vi "S2C_FORNAX_Proc_Open.vi"(8 "Error In":errorcluster, 10 "Timeout":dbl, 11 "Data":string) -> (0 "Error Out":errorcluster, 3 "FXN_Ref":refnum<k5>)   [LabVIEW 2015]
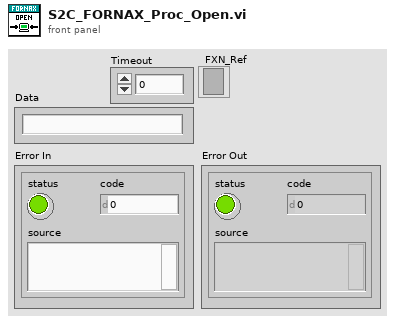
[diagram p1: front panel]
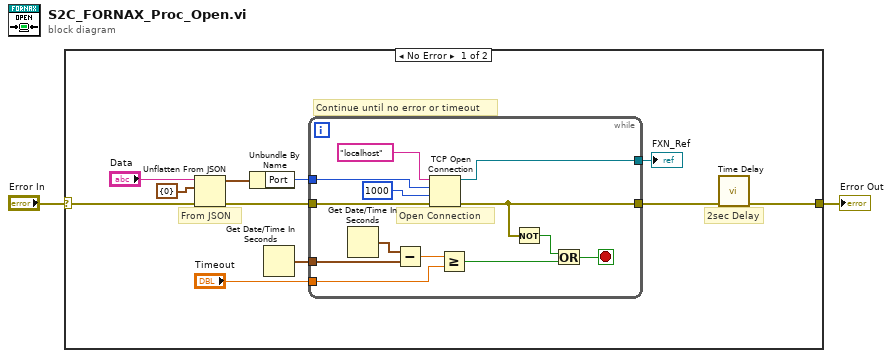
[diagram p0: block diagram]
diagram:
  n1 = case shown="No Error" "Error In" {
    selector: "Error In" -> [w6 w27]
    tunnel: [w9 w27] -> w1
    frame No Error {
      # "From JSON"
      # "2sec Delay"
      # "Continue until no error or timeout"
      n2 = Unflatten From JSON(JSON string="Data", type and defaults=cluster{"Port":u16} {"Port"=0} ("Feature Set"), error in (no error)=w6) -> (value=w7:cluster{"Port":u16}, error out=w5:errorcluster)  [unwired: 4 in]
      n3 = Unbundle By Name(w7) -> ("Port"=w4:u16)
      n4 = Get Date/Time In Seconds() -> (seconds since 1Jan1904=w13:timestamp)
      n5 = while {
        tunnel: [w24] -> w11
        tunnel: w13 -> [w20]
        tunnel: "Timeout" -> [w19]
        tunnel: w5 -> [w23]
        tunnel: [w15] -> w10
        tunnel: w4 -> [w14]
        stop <- w16 stop-if-true
        # "Open Connection"
        n6 = Get Date/Time In Seconds() -> (seconds since 1Jan1904=w21:timestamp)
        n7 = Subtract(x=w21, y=w20) -> (x-y=w22:dbl)
        n8 = TCP Open Connection(address="localhost", remote port or service name=w14, timeout ms (60000)=1000 ("timeout ms (wait forever: -1)"), error in (no error)=w23) -> (connection ID=w24:refnum<k5>, error out=w15:errorcluster)  [unwired: 1 in]
        n9 = Greater Or Equal?(x=w22, y=w19) -> (x >= y?=w17:bool)
        n10 = Not(x=w15) -> (.not. x?=w18:bool)
        n11 = Or(x=w18, y=w17) -> (x .or. y?=w16:bool)
      }
      "FXN_Ref" <- w11
      n12 = call "Time Delay"("error in (no error)"=w10) -> ("error out"=w9:errorcluster)  [unwired: 10 in]
    }
    frame Error {
    }
  }
  "Error Out" <- w1
